vi "Dequeue Message.vi"(8 "error in (no error)":T1 caption="entrée d'erreur (pas d'erreur)", 11 "File d'attente de messages":refnum<queue>) -> (0 "error out":T1 caption="sortie d'erreur", 1 "Données de message":variant, 2 "Message":string, 3 "File d'attente de message dup.":refnum<queue>)   [LabVIEW 2020, in "Message Queue.lvlib"]
doc: "Ce VI extrait des messages de la file d'attente de messages."
uses:
  Message Queue.lvlib
  Message Cluster.ctl
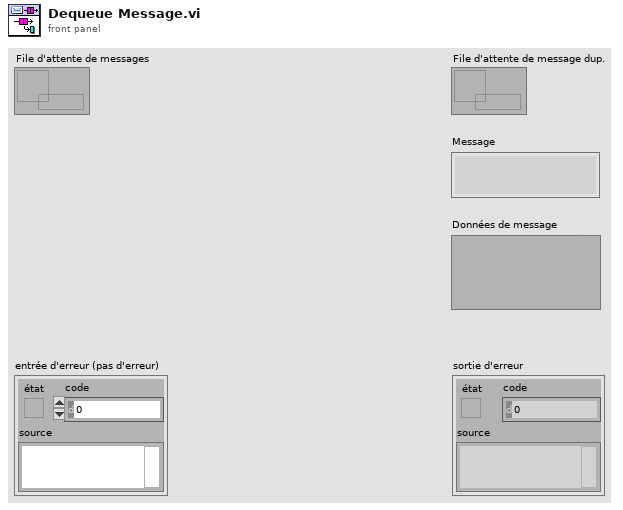
[diagram p1: front panel]
types:
  T1 = cluster{"état":bool, "code":i32, "source":string}
  T2 = typedef "Message Queue.lvlib/Message Cluster.ctl" = cluster{"Message":string, "Données de message":variant}
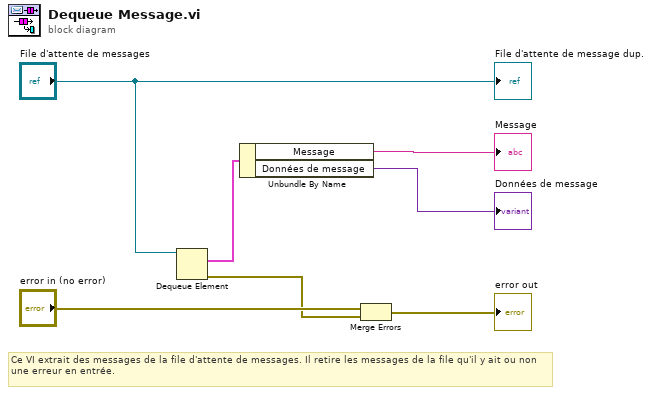
[diagram p0: block diagram]
diagram:
  # "Ce VI extrait des messages de la file d'attente de messages. Il retire les messages de la file qu'il y ait ou non une erreur en entrée."
  n1 = Dequeue Element(queue="File d'attente de messages") -> (element=w4:T2, error out=w1:errorcluster)  [unwired: 2 in, 2 out]
  n2 = Unbundle By Name(w4) -> ("Message"=→"Message":string, "Données de message"=→"Données de message":variant)
  n3 = Merge Errors("error in (no error)", w1) -> (→"error out":errorcluster)
  "File d'attente de message dup." <- "File d'attente de messages"
